vi "Create Gradient Color by Segment.vi"(8 "错误输入":errorcluster, 10 "Length":i32=256, 11 "Color Segement":u32[](array[colorbox])=[16448250, 0, 16736786, 1198079]) -> (0 "错误输出":errorcluster, 2 "1 Pix W - Color Box Array":u32[](array[colorbox])=[14277081, 14145495, 13948116, 13816530, 13619151, 13487565, 13290186, 13092807, 12961221, 12763842, 12632256, 12434877, 12303291, 12105912, 11974326, 11776947, 11645361, 11447982, 11316396, 11119017, 10987431, 10790052, 10658466, 10461087, 10329501, 10132122, 10000536, 9803157, 9605778, 9474192, 9276813, 9145227, 8947848, 8816262, 8618883, 8487297, 8289918, 8158332, 7960953, 7829367, 7631988, 7500402, 7303023, 7171437, 6974058, 6842472, 6645093, 6447714, 6316128, 6118749, 5987163, 5789784, 5658198, 5460819, 5329233, 5131854, 5000268, 4802889, 4671303, 4473924, 4342338, 4144959, 4013373, 3815994, 3684408, 3487029, 3355443, 3158064, 2960685, 2829099, 2631720, 2500134, 2302755, 2171169, 1973790, 1842204, 1644825, 1513239, 1315860, 1184274, 986895, 855309, 657930, 526344, 328965, 197379, 0, 0, 197379, 328965, 526344, 657930, 855309, 986895, 1184274, 1315860, 1513239, 1644825, 1842204, 1973790, 2171169, 2302755, 2500134, 2631720, 2829099, 2960685, 3158064, 3355443, 3487029, 3684408, 3815994, 4013373, 4144959, 4342338, 4473924, 4671303, 4802889, 5000268, 5131854, 5329233, 5460819, 5658198, 5789784, 5987163, 6118749, 6316128, 6447714, 6645093, 6842472, 6974058, 7171437, 7303023, 7500402, 7631988, 7829367, 7960953, 8158332, 8289918, 8487297, 8618883, 8816262, 8947848, 9145227, 9276813, 9474192, 9605778, 9803157, 10000536, 10132122, 10329501, 10461087, 10658466, 10790052, 10987431, 11119017, 11316396, 11447982, 11645361, 11776947, 11974326, 12105912, 12303291, 12434877, 12632256, 12763842, 12961221, 13092807, 13290186, 13487565, 13619151, 13816530, 13948116, 14145495, 14277081, 14474460, 14606046, 14803425, 14935011, 15132390, 15263976, 15461355, 15592941, 15790320, 15921906, 16119285, 16250871, 16448250, 16448250, 16250871, 16119285, 15921906, 15790320, 15592941, 15461355, 15263976, 15132390, 14935011, 14803425, 14606046, 14474460], 3 "1 Pix H - Color Box Array":u32[](array[colorbox]))   [LabVIEW 2012, in "Picture Box Tools.lvlib"]
uses:
  Picture Box Tools.lvlib
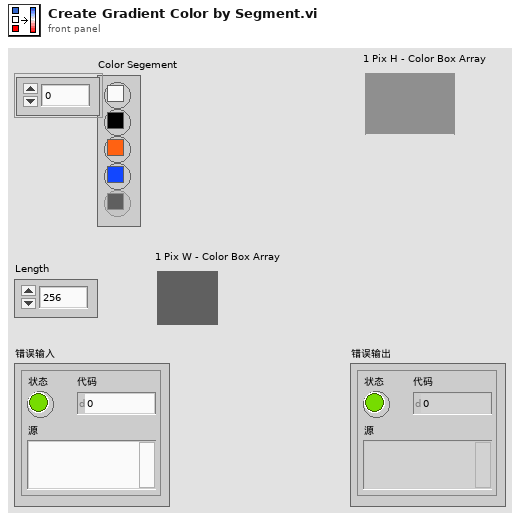
[diagram p1: front panel]
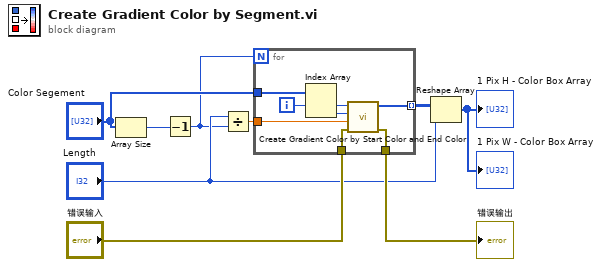
[diagram p0: block diagram]
diagram:
  n1 = Array Size(array="Color Segement") -> (size(s)=w9:i32)
  n2 = Decrement(x=w9) -> (x-1=w2:i32)
  n3 = Divide(x="Length", y=w2) -> (x/y=w1:dbl)
  n4 = for {
    N: w2 -> [_]
    tunnel: w1 -> [w17]
    tunnel: "Color Segement" -> [w15]
    tunnel: [w12] -> w7 mode=indexing
    tunnel: "错误输入" -> [w11]
    tunnel: [w10] -> w5
    i -> [w16]
    n5 = Index Array(array=w15, index #1=w16) -> (element #1=w14:u32, element #2=w13:u32)  [unwired: 1 in]
    n6 = call "Create Gradient Color by Start Color and End Color.vi"("错误输入"=w11, "Length"=w17, "End"=w13, "Start"=w14) -> ("错误输出"=w10:errorcluster, "ColorArray"=w12:u32[])  [unwired: 6 in]
  }
  "错误输出" <- w5
  n7 = Reshape Array(w7, "Length") -> (→"1 Pix H - Color Box Array" →"1 Pix W - Color Box Array":u32[])
